vi "niusrprios Write FIFO (Multi-Channel).vi"(0 "data in":u32[](array[numeric])=[0, 0], 1 "reset":bool, 2 "FIFO 0":refnum<k21>, 3 "FIFO 1":refnum<k21>, 5 "enabled":bool[](array[boolean])=[FALSE, FALSE], 9 "input valid":bool) -> (14 "ready for input":bool)   [LabVIEW 2015]
doc: "Writes data to multiple 32-bit FIFOs. This VI is a wrapper around the LabVIEW FPGA FIFO Write method. This VI exposes handshaking signals that inform the user when the FIFOs are ready to accept new data.\n\n<B>Input Parameters</B>\n\n<B>data in</B> is the data to be written to the FIFO.\n\n<B>enabled</B> specifies which streams are enabled.\n\n<B>input valid</B> specifies when 'data in' is valid.\n\n<B>reset</B> the LabVIEW FPGA FIFO.\n\n<B>FIFO 0</B> is the reference to the FIFO to which data received on channel 0 will be written to.\n\n<B>FIFO 1</B> is the reference to the FIFO to which data received on channel 1 will be written to.\n\n<B>Output Parameters</B>\n\n<B>ready for input</B> is a flow control signal that indicates whether the Write FIFO VI is ready to accept new data."
uses:
  <instrlib>/_niInstr/Basic Elements/v1/FPGA/Private/Write U32 FIFO.vi
  <instrlib>/_niInstr/Basic Elements/v1/FPGA/niInstr Basic Elements v1 FPGA.lvlib
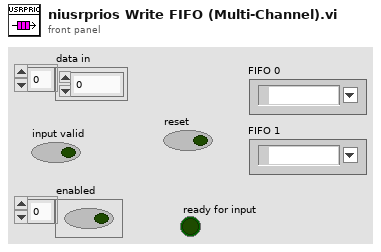
[diagram p1: front panel]
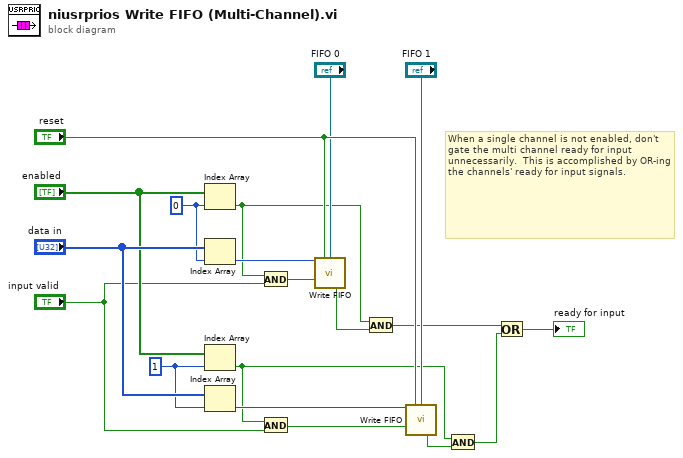
[diagram p0: block diagram]
diagram:
  w15 = 1 ("index")
  w17 = 0 ("index")
  # "When a single channel is not enabled, don't gate the multi channel ready for input unnecessarily.  This is accomplished by OR-ing the channels' ready for input signals."
  n1 = Index Array(array="enabled", index=w17) -> (element=w4:bool)
  n2 = Index Array(array="data in", index=w17) -> (element=w18:u32)
  n3 = Index Array(array="enabled", index=w15) -> (element=w3:bool)
  n4 = Index Array(array="data in", index=w15) -> (element=w12:u32)
  n5 = And(x=w4, y="input valid") -> (x .and. y?=w16:bool)
  n6 = And(x=w3, y="input valid") -> (x .and. y?=w13:bool)
  n7 = call-poly <instrlib>:"Write FIFO.vi"("input data"=w18, "reset"="reset", "fifo"="FIFO 0", "input valid"=w16) -> ("ready for input"=w2:bool)  [unwired: 11 in]
  n8 = And(x=w4, y=w2) -> (x .and. y?=w5:bool)
  n9 = call-poly <instrlib>:"Write FIFO.vi"("input data"=w12, "reset"="reset", "fifo"="FIFO 1", "input valid"=w13) -> ("ready for input"=w1:bool)  [unwired: 11 in]
  n10 = And(x=w3, y=w1) -> (x .and. y?=w6:bool)
  n11 = Or(x=w5, y=w6) -> (x .or. y?=→"ready for input":bool)
